vi "File整体图.vi"() -> ()   [LabVIEW 2014]
panel:
  in  "New file":bool
  in  "Floppy":bool
  in  "Find":bool
  in  "Export file":bool
  in  "Diskette":bool
  in  "Close file":bool
  in  "Word":bool
  in  "Save oo":bool
  in  "Save file":bool
  in  "Save file as":bool
  in  "Save all":bool
  in  "Revert":bool
  in  "Open office":bool
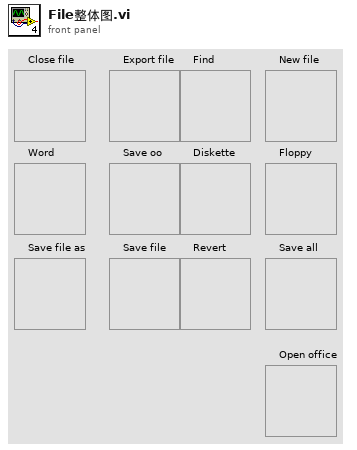
[diagram p1: front panel]
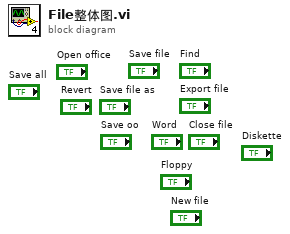
[diagram p0: block diagram]
diagram:
